vi "ClimatronicsUDP_get_rdg.vi"(4 "Channel Name":string, 7 "Address":T1={"Main"=61557, "Ch."=0, "Sub"=982, "Port Name"=""}) -> (0 "Output":dbl format="%.2f", 3 "Status note":string)   [LabVIEW 2015]
uses:
  ADAM Client/Sub VIs/ADAM Controls/Address.ctl
  ADAM Client/Sub VIs/ADAM Controls/Remember_value_mode.ctl
panel:
  out "UDPopenError":errorcluster
  out "UDPreadError":errorcluster
  # "Channels:\n0: Velocity\n1: Direction\n2: Northerly\n3: Easterly\n4: Supply Volts\n5: 999Error\n6: ParseError\n7: SerialNo"
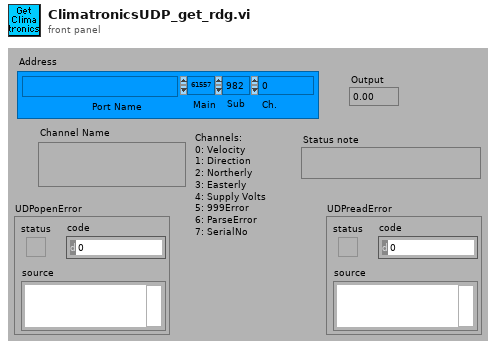
[diagram p1: front panel]
types:
  T1 = typedef "Address.ctl" = cluster{"Main":i32, "Ch.":i32, "Sub":i32, "Port Name":string}
  T2 = typedef "Remember_value_mode.ctl" = enum16{"Read only", "Read and Write"}
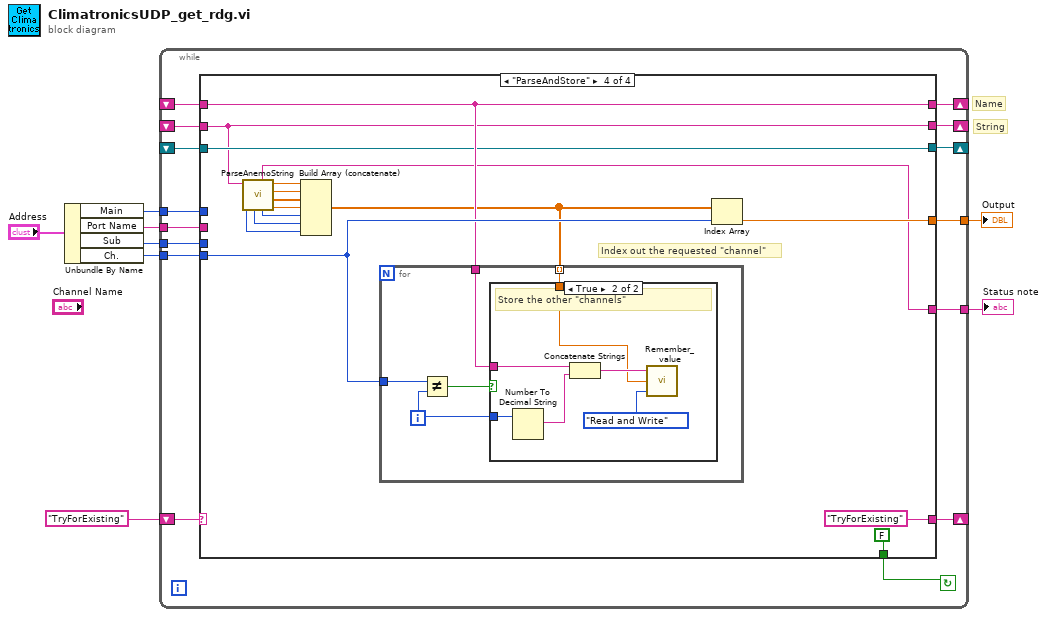
[diagram p0: block diagram]
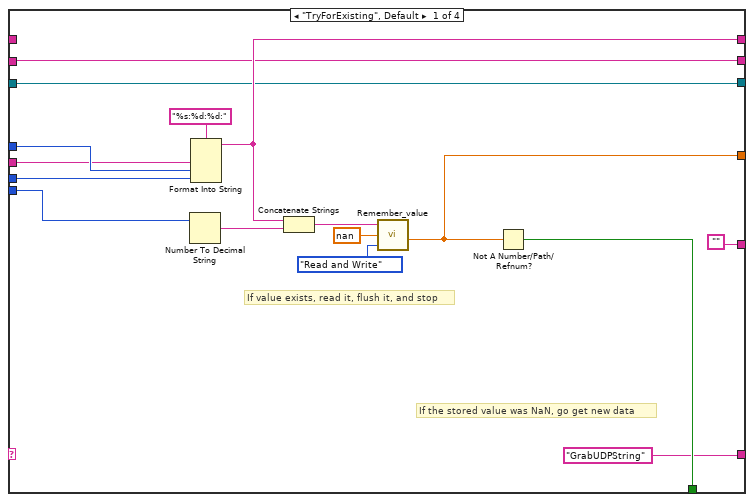
[diagram p2: hidden frame]
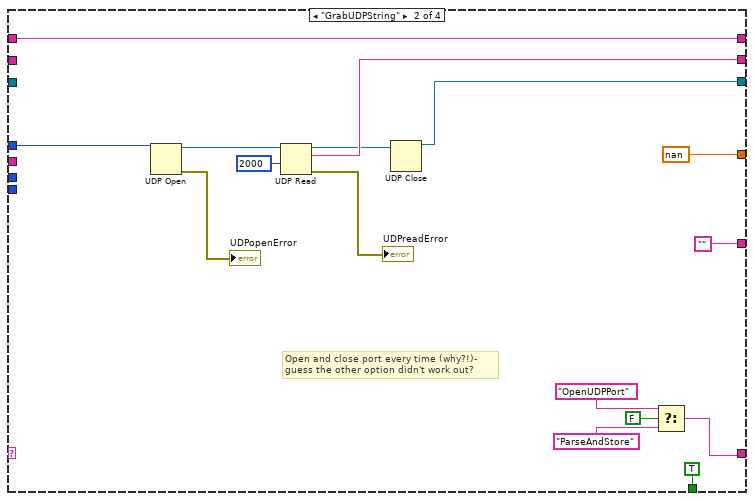
[diagram p3: hidden frame]
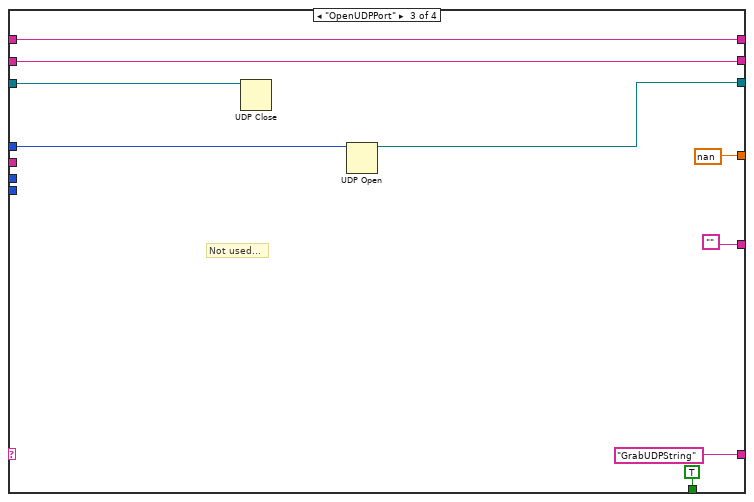
[diagram p4: hidden frame]
diagram:
  # "String"
  # "Name"
  n1 = Unbundle By Name("Address") -> ("Main"=w2:i32, "Port Name"=w7:string, "Sub"=w6:i32, "Ch."=w3:i32)
  n2 = while {
    shift-left: _ -> [w11]
    shift-right: [w12] -> _
    shift-left: _ -> [w14]
    shift-right: [w15] -> _
    tunnel: [w17] -> w4
    tunnel: [w18] -> w5
    shift-left: _ -> [w13]
    shift-right: [w19] -> _
    shift-left: "TryForExisting" -> [w10]
    shift-right: [w9] -> _
    tunnel: w3 -> [w20]
    tunnel: w2 -> [w21]
    tunnel: w6 -> [w22]
    tunnel: w7 -> [w23]
    stop <- w16 continue-if-true
    n3 = case shown="\"ParseAndStore\"" w10 {
      tunnel: w23 -> [w26 _ _ _]
      tunnel: w22 -> [w38 _ _ _]
      tunnel: w21 -> [w39 w46 w62 _]
      tunnel: w20 -> [w36 _ _ w78]
      tunnel: ["GrabUDPString" w49 "GrabUDPString" "TryForExisting"] -> w9
      tunnel: [w35 w54 w60 w77] -> w19
      tunnel: [w28 nan nan w79] -> w18
      tunnel: ["" "" "" w65] -> w17
      tunnel: [w27 TRUE TRUE FALSE] -> w16
      tunnel: [w30 w53 w59 w75] -> w15
      tunnel: w14 -> [w30 _ w59 w75]
      tunnel: w13 -> [_ w54 w60 w77]
      tunnel: [w25 w40 w64 w76] -> w12
      tunnel: w11 -> [w25 _ w63 w76]
      frame "TryForExisting", Default {
        # "If the stored value was NaN, go get new data"
        # "If value exists, read it, flush it, and stop"
        n4 = Number To Decimal String(number=w36) -> (decimal integer string=w34:string)  [unwired: 1 out]
        n5 = Format Into String(format string="%s:%d:%d:" ("Format String"), w26, w39, w38) -> (resulting string=w35:string)  [unwired: 2 in, 1 out]
        n6 = Concatenate Strings(w35, w34) -> (w33:string)
        n7 = call "Remember_value.vi"("Mode"=Remember_value_mode."Read and Write", "Input Value"=nan, "Ch name"=w33) -> ("Output Value"=w28:dbl)
        n8 = Not A Number/Path/Refnum?(number/path/refnum=w28) -> (NaN/Path/Refnum?=w27:bool)
      }
      frame "GrabUDPString" {
        # "Open and close port every time (why?!)-\nguess the other option didn't work out?"
        n9 = UDP Open(11:w46) -> (port=w45:refnum<k16>, 0:→"UDPopenError":errorcluster)  [unwired: 4 in, 1 out]
        n10 = UDP Read(connection ID=w45, timeout ms (25000)=2000) -> (data out=w53:string, error out=→"UDPreadError":errorcluster, 3:w41:refnum<k16>)  [unwired: 2 in, 2 out]
        n11 = UDP Close(connection ID=w41) -> (connection ID out=w40:refnum<k16>)  [unwired: 1 in, 1 out]
        n12 = Select(t="OpenUDPPort", s=FALSE, f="ParseAndStore") -> (s? t:f=w49:string)
      }
      frame "OpenUDPPort" {
        # "Not used..."
        n13 = UDP Close(connection ID=w63) -> ()  [unwired: 1 in, 2 out]
        n14 = UDP Open(11:w62) -> (port=w64:refnum<k16>)  [unwired: 4 in, 2 out]
      }
      frame "ParseAndStore" {
        # "Index out the requested \"channel\""
        n15 = call "ParseAnemoString.vi"("String"=w75) -> ("SupplyVolts"=w69:dbl, "N,E Components"=w70:dbl[], "direction"=w72:dbl, "speed"=w73:dbl, "999Error"=w68:i32, "Status"=w65:string, "ParseError"=w67:i32, "SerialNo"=w66:i32)  [unwired: 3 in]
        n16 = Build Array (concatenate)(w73, w72, w70, w69, w68, w67, w66) -> (w71:dbl[])
        n17 = for {
          tunnel: w77 -> [w85]
          tunnel: w71 -> [w84] mode=indexing
          tunnel: w78 -> [w82]
          i -> [w83]
          n18 = Not Equal?(x=w82, y=w83) -> (x != y?=w81:bool)
          n19 = case shown="True" w81 {
            tunnel: w83 -> [_ w91]
            tunnel: w85 -> [_ w89]
            tunnel: w84 -> [_ w86]
            frame False {
              # "Don't store the requested channel"
            }
            frame True {
              # "Store the other \"channels\""
              n20 = Number To Decimal String(number=w91) -> (decimal integer string=w90:string)  [unwired: 1 out]
              n21 = Concatenate Strings(w89, w90) -> (w87:string)
              n22 = call "Remember_value.vi"("Mode"=Remember_value_mode."Read and Write", "Input Value"=w86, "Ch name"=w87) -> ()  [unwired: 1 out]
            }
          }
        }
        n23 = Index Array(array=w71, index=w78) -> (element=w79:dbl)
      }
    }
  }
  "Output" <- w5
  "Status note" <- w4
